vi "DSKNM.vi"() -> ()   [LabVIEW 2023]
panel:
  in  "stop":bool
  out "min index":i32
  out "minDate":string[](array[string])
  out "Min":dbl format="%#_5g"
  out "Max":dbl
  out "All Sum":dbl
  out "Transfer numbers":i32
  out "maxDate":string[](array[string])
  out "tmpArr":string[][](array[string])
  out "Waveform Chart":i32(graph)
  out "TableRes":string[][](table)
  in  "Transaction Type":T1(ring)
  in  "file path":path
  # "$"
  # "$"
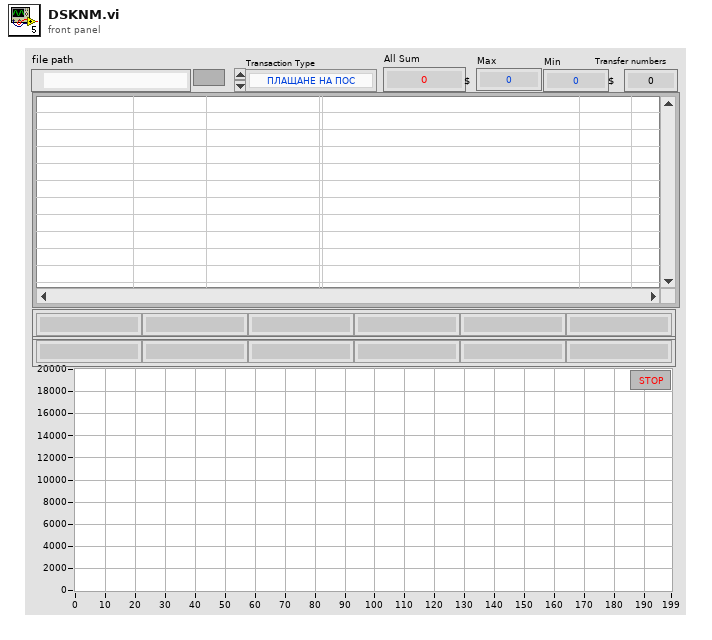
[diagram p1: front panel]
types:
  T1 = enum16{"ПЛАЩАНЕ НА ПОС", "СБКО", "ТЕГЛЕНЕ", "ЗАЕМ", "BREZOVO", "VIVACOM", "ЕЛЕКТРОХОЛД", "ЕВН", "ЗАПЛАТА", "АВАНС", "НЕТ", "ТРАНСФЕР"}
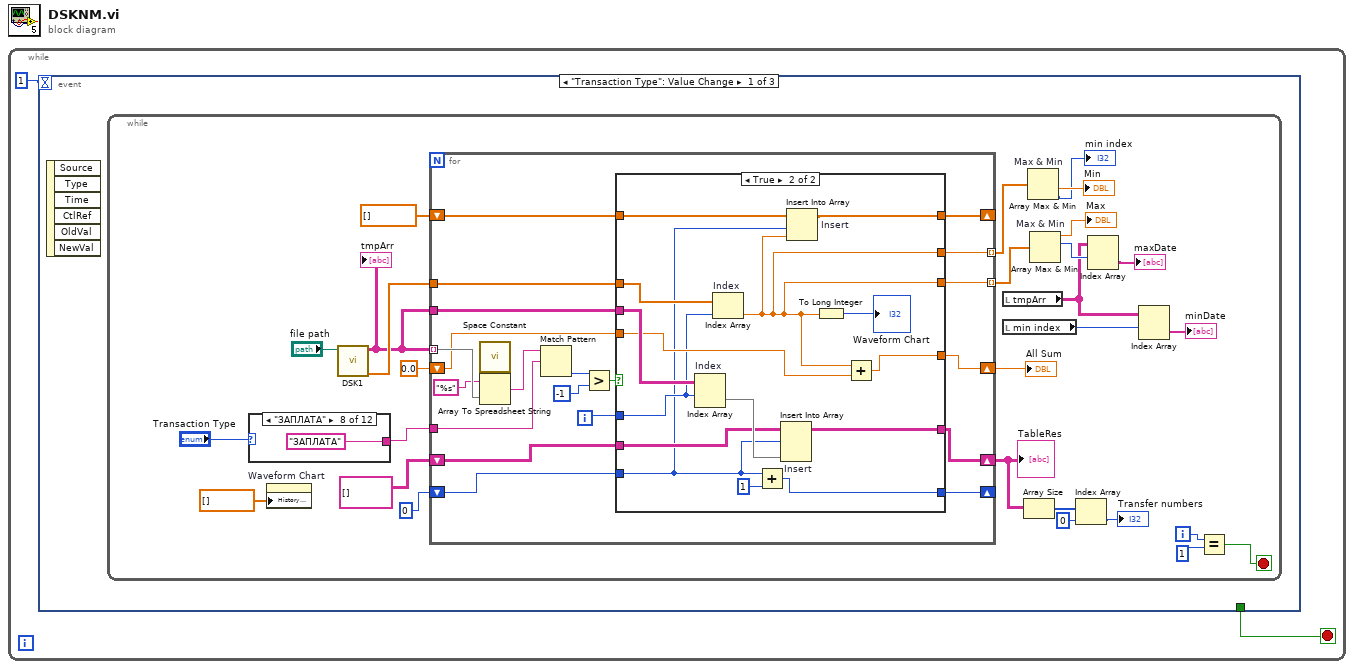
[diagram p0: block diagram]
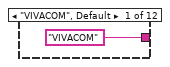
[diagram p2: hidden frame]
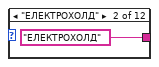
[diagram p3: hidden frame]
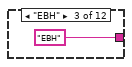
[diagram p4: hidden frame]
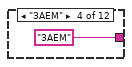
[diagram p5: hidden frame]
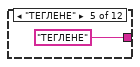
[diagram p6: hidden frame]
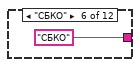
[diagram p7: hidden frame]
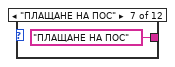
[diagram p8: hidden frame]
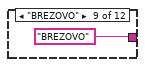
[diagram p9: hidden frame]
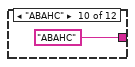
[diagram p10: hidden frame]
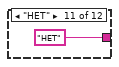
[diagram p11: hidden frame]
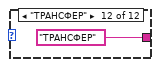
[diagram p12: hidden frame]
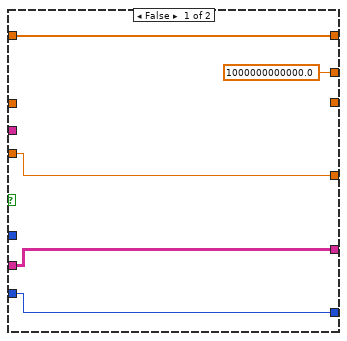
[diagram p13: hidden frame]
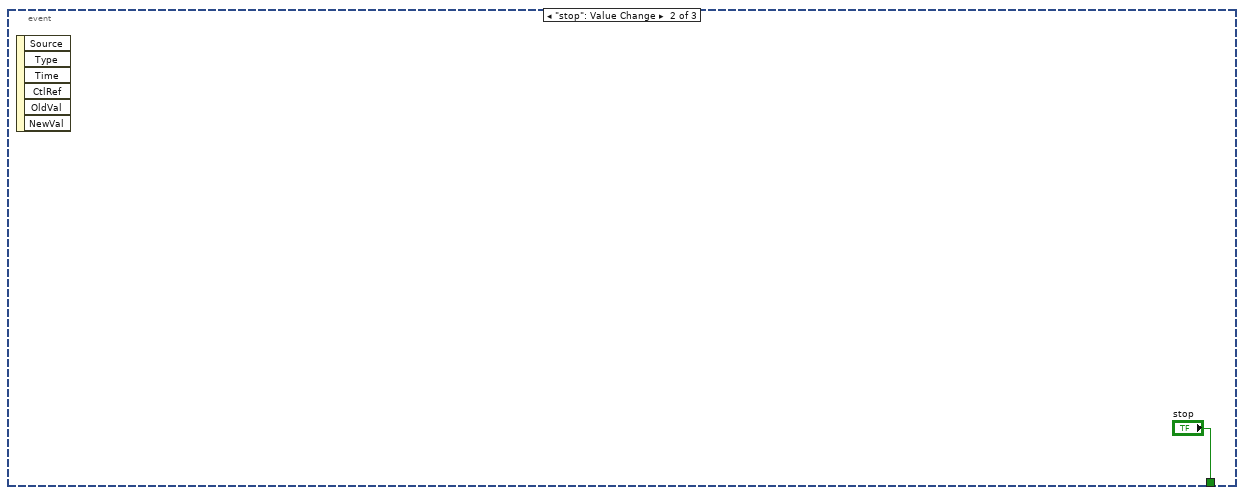
[diagram p14: hidden frame]
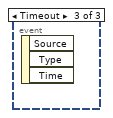
[diagram p15: hidden frame]
diagram:
  n1 = while {
    stop <- w2 stop-if-true
    n2 = event shown="[0] \"Transaction Type\": Value Change" {
      selector: _ -> [_ _ _]
      dyn-events: _ -> [_ _ _]
      timeout: 1 -> [_ _ _]
      tunnel: [_ "stop" _] -> w2
      event "Transaction Type": Value Change {
        n3 = event-data() -> ()  [unwired: 1 in, 6 out]
        n4 = while {
          i -> [w6]
          stop <- w4 stop-if-true
          n5 = case shown="\"ЗАПЛАТА\"" "Transaction Type" {
            tunnel: ["VIVACOM" "ЕЛЕКТРОХОЛД" "ЕВН" "ЗАЕМ" "ТЕГЛЕНЕ" "СБКО" "ПЛАЩАНЕ НА ПОС" "ЗАПЛАТА" "BREZOVO" "АВАНС" "НЕТ" "ТРАНСФЕР"] -> w28
            frame "VIVACOM", Default {
            }
            frame "ЕЛЕКТРОХОЛД" {
            }
            frame "ЕВН" {
            }
            frame "ЗАЕМ" {
            }
            frame "ТЕГЛЕНЕ" {
            }
            frame "СБКО" {
            }
            frame "ПЛАЩАНЕ НА ПОС" {
            }
            frame "ЗАПЛАТА" {
            }
            frame "BREZOVO" {
            }
            frame "АВАНС" {
            }
            frame "НЕТ" {
            }
            frame "ТРАНСФЕР" {
            }
          }
          n6 = property on="Waveform Chart" class="WFChart (strict)"("History Data"=dbl[] []) -> ()  [unwired: 2 in, 2 out]
          n7 = call "DSK1.vi"("file path (dialog if empty)"="file path") -> ("Money"=w15:dbl[], "Transfers"=w13:string[][])  [unwired: 9 in]
          "tmpArr" <- w13
          n8 = for {
            tunnel: w13 -> [w55] mode=indexing
            tunnel: w28 -> [w56]
            tunnel: w13 -> [w62]
            shift-right: [w59] -> _
            shift-left: 0 -> [w60]
            shift-right: [w58] -> w24
            shift-left: string[][] [] -> [w57]
            tunnel: w15 -> [w49]
            shift-right: [w47] -> w20
            shift-left: 0.0 -> [w48]
            shift-right: [w46] -> _
            shift-left: dbl[] [] -> [w45]
            tunnel: [w44] -> w16 mode=indexing
            tunnel: [w43] -> w10 mode=indexing
            i -> [w61]
            n9 = call <vilib>:"Space Constant.vi"() -> ("String"=w54:string)
            n10 = Array To Spreadsheet String(delimiter (Tab)=w54, array=w55, 3:"%s" ("format string")) -> (spreadsheet string=w53:string)
            n11 = Match Pattern(string=w53, regular expression=w56) -> (offset past match=w50:i32)  [unwired: 1 in, 3 out]
            n12 = Greater?(x=w50, y=-1) -> (0:w63:bool)
            n13 = case shown="True" w63 {
              tunnel: w62 -> [_ w83]
              tunnel: w61 -> [_ w74]
              tunnel: w60 -> [w67 w71]
              tunnel: [w67 w81] -> w59
              tunnel: [w68 w80] -> w58
              tunnel: w57 -> [w68 w78]
              tunnel: w49 -> [_ w75]
              tunnel: [w66 w77] -> w47
              tunnel: w48 -> [w66 w76]
              tunnel: [w65 w73] -> w46
              tunnel: w45 -> [w65 w72]
              tunnel: [_ w70] -> w44
              tunnel: [1000000000000.0 w70] -> w43
              frame False {
              }
              frame True {
                n14 = Index Array "Index"(array=w83, index (row)=w74) -> (element=w79:string[])  [unwired: 1 in]
                n15 = Index Array "Index"(array=w75, index=w74) -> (element=w70:dbl)
                n16 = Add(x=w71, y=1) -> (x+y=w81:i32)
                n17 = Insert Into Array "Insert"(array=w78, index (row)=w71, new element=w79) -> (w80:string[][])  [unwired: 1 in]
                n18 = Insert Into Array "Insert"(array=w72, index=w71, new element=w70) -> (w73:dbl[])
                n19 = To Long Integer(number=w70) -> (32bit integer=→"Waveform Chart":i32)
                n20 = Add(x=w70, y=w76) -> (x+y=w77:dbl)
              }
            }
          }
          "All Sum" <- w20
          "TableRes" <- w24
          n21 = local read "tmpArr"() -> (w3:string[][])
          n22 = local read "min index"() -> (w7:i32)
          n23 = Array Size(array=w24) -> (size(s)=w23:i32[])
          n24 = Array Max & Min "Max & Min"(array=w10) -> (min value=→"Min":dbl, min index (indices)=→"min index":i32)  [unwired: 2 out]
          n25 = Array Max & Min "Max & Min"(array=w16) -> (max value=→"Max":dbl, max index (indices)=w14:i32)  [unwired: 2 out]
          n26 = Index Array(array=w23, index=0) -> (element=→"Transfer numbers":i32)
          n27 = Index Array(array=w3, index (row)=w14) -> (element=→"maxDate":string[])  [unwired: 1 in]
          n28 = Index Array(array=w3, index (row)=w7) -> (element=→"minDate":string[])  [unwired: 1 in]
          n29 = Equal?(x=w6, y=1) -> (x = y?=w4:bool)
        }
      }
      event "stop": Value Change {
        n30 = event-data() -> ()  [unwired: 1 in, 6 out]
      }
      event Timeout {
        n31 = event-data() -> ()  [unwired: 1 in, 3 out]
      }
    }
  }
